vi "Write_parameter.vi"(8 "error in (no error)":errorcluster caption="entrée d'erreur (pas d'erreur)", 10 "Parameter":string, 11 "Class Relay_Board en entrée":refnum<class "Class Instrument Relay_Board.lvclass">) -> (0 "error out":errorcluster caption="sortie d'erreur", 3 "Class Relay_Board en Sortie":refnum<class "Class Instrument Relay_Board.lvclass">)   [LabVIEW 2020, in "Library Instrument & Equipement.lvlib" / "Library Instruments.lvlib" / "Class Instrument Relay_Board.lvclass"]
uses:
  Class Instrument Relay_Board.lvclass
  Commun VI/TypeDef/Commande Relay_Board/Parameter Relay_Board.ctl
  Relay_Board/Relay_Board (Default)/Class Relay_Board (Default).lvclass
  JSON API/JSON Value/Set from JSON string.vi
  Instrument (Default)/Class Instrument (Default).lvclass
  JSON API/JSON Value/JSON Value.lvclass
  Class Instrument Relay_Board.lvclass/Class Instrument Relay_Board.ctl
  JSON API/Variant JSON/Variant JSON.lvlib
  JSON API/Get Polymorphic/JSON GetSet.lvlib
  Commun VI/Library Commun.lvlib
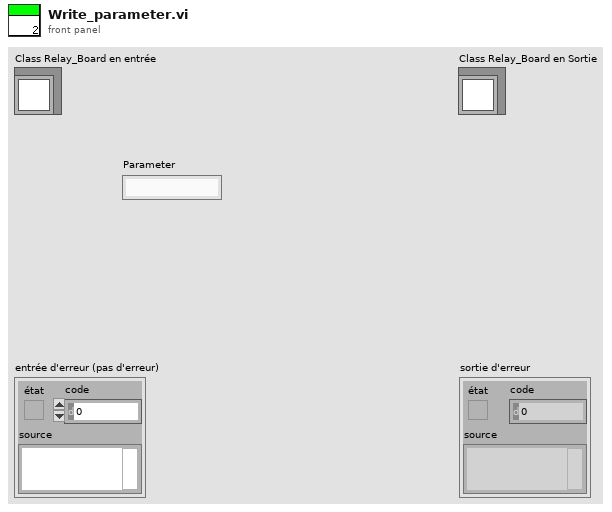
[diagram p1: front panel]
types:
  T1 = typedef "Library Commun.lvlib/Parameter Relay_Board.ctl" = cluster{"Device_Com_Port":string, "Address Board":string, "Tab_Num_Relay":u8[], "Parameter Class Relay_Board":refnum<class "Class Relay_Board (Default).lvclass">}
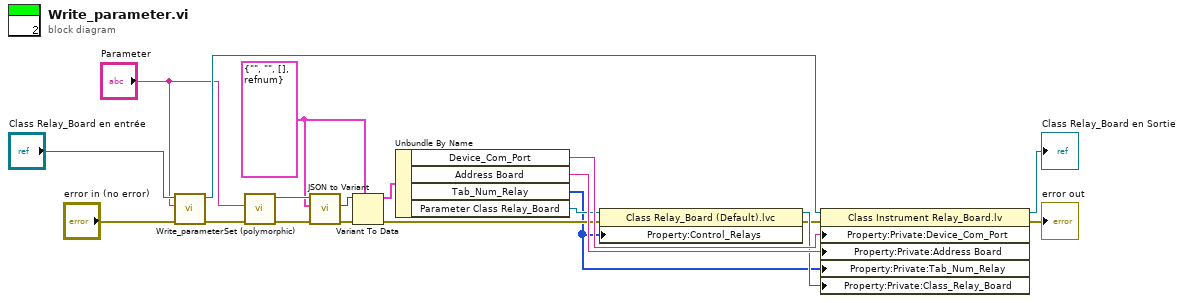
[diagram p0: block diagram]
diagram:
  w10 = T1 {"Device_Com_Port"="", "Address Board"="", "Tab_Num_Relay"=[], "Parameter Class Relay_Board"=refnum} ("Parameter")
  n1 = call-parent "Write_parameter.vi"("error in (no error)"="error in (no error)", "Parameter"="Parameter", "Class Instrument (Default) en entrée"="Class Relay_Board en entrée") -> ("error out"=w9:errorcluster, "Class Instrument (Default) en sortie"=w7:refnum<class "Class Instrument Relay_Board.lvclass">)  [unwired: 7 in]
  n2 = call-poly "Set (polymorphic).vi"("error in (no error)"=w9, "JSON stream"="Parameter") -> ("error out"=w18:errorcluster, "JSON Value out"=w20:refnum<class "JSON Value.lvclass">)  [unwired: 7 in, 1 out]
  n3 = call "JSON to Variant.vi"("error in (no error)"=w18, "Variant (Data Type)"=w10, "JSON Value"=w20) -> ("error out"=w19:errorcluster, "Variant out"=w17:variant)  [unwired: 7 in]
  n4 = Variant To Data(error in=w19, type=w10, Variant=w17) -> (data=w13:T1, error out=w3:errorcluster)
  n5 = Unbundle By Name(w13) -> ("Device_Com_Port"=w11:string, "Address Board"=w12:string, "Tab_Num_Relay"=w1:u8[], "Parameter Class Relay_Board"=w5:refnum<class "Class Relay_Board (Default).lvclass">)
  n6 = property class="Class Relay_Board (Default).lvc"(reference=w5, error in=w3, "Property:Control_Relays"=w1) -> (reference out=w4:refnum<class "Class Relay_Board (Default).lvclass">, error out=w2:errorcluster)
  n7 = property class="Class Instrument Relay_Board.lv"(reference=w7, error in=w2, "Property:Private:Device_Com_Port"=w11, "Property:Private:Address Board"=w12, "Property:Private:Tab_Num_Relay"=w1, "Property:Private:Class_Relay_Board"=w4) -> (reference out=→"Class Relay_Board en Sortie":refnum<class "Class Instrument Relay_Board.lvclass">, error out=→"error out":errorcluster)
